vi "writeMessage.vi"(8 "error in (no error)":errorcluster, 10 "Message":string, 11 "CSVTestLog in":refnum<class "CSVTestLog.lvclass">) -> (0 "error out":errorcluster, 3 "CSVTestLog out":refnum<class "CSVTestLog.lvclass">)   [LabVIEW 2015, in "CSVTestLog.lvclass"]
uses:
  CSVTestLog.lvclass
  CSVTestLog.lvclass/CSVTestLog.ctl
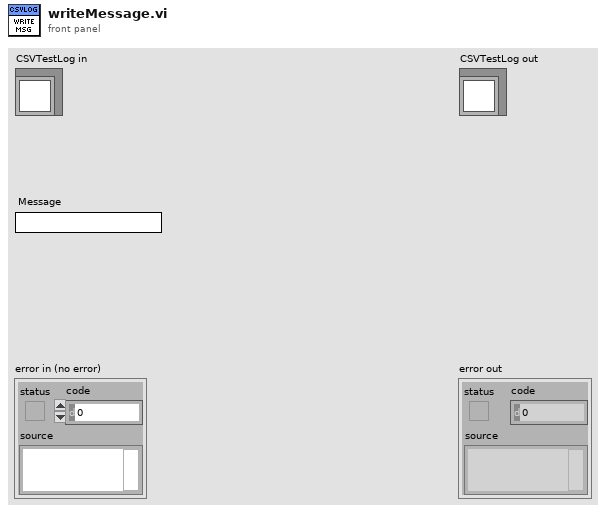
[diagram p1: front panel]
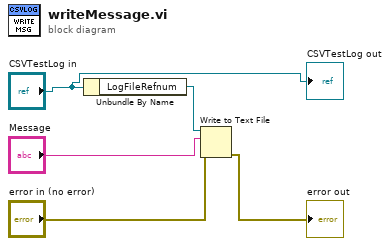
[diagram p0: block diagram]
diagram:
  n1 = Unbundle By Name("CSVTestLog in") -> ("LogFileRefnum"=w5:refnum<file>)
  n2 = Write to Text File(file (use dialog)=w5, text="Message", error in="error in (no error)") -> (error out=→"error out":errorcluster)  [unwired: 1 in, 2 out]
  "CSVTestLog out" <- "CSVTestLog in"
